vi "FileIO - Save ROI Results.vi"(11 "ROI Results":T1(array[cluster])) -> ()   [LabVIEW 2014]
uses:
  TypeDef - File Actions.ctl
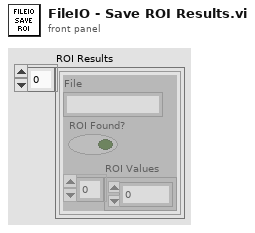
[diagram p1: front panel]
types:
  T1 = cluster{"File":string, "ROI Found?":bool, "ROI Values":dbl[]}[]
  T2 = typedef "TypeDef - File Actions.ctl" = enum16{"Read", "Write", "Get Current"}
  T3 = typedef "TypeDef - System Configuration.ctl" = cluster{"Results FilePath":path, "Analysis Parameters":cluster{"Area":cluster{"Lower Value":dbl, "Upper Value":dbl}, "Circle Filter Radius":cluster{"Lower Value":sgl, "Upper Value":sgl}, "Edge Detection Threshold":u16}, "ROI Parameters":cluster{"ROI size (in Radius)":cluster{"Width":dbl, "Height":dbl}}}
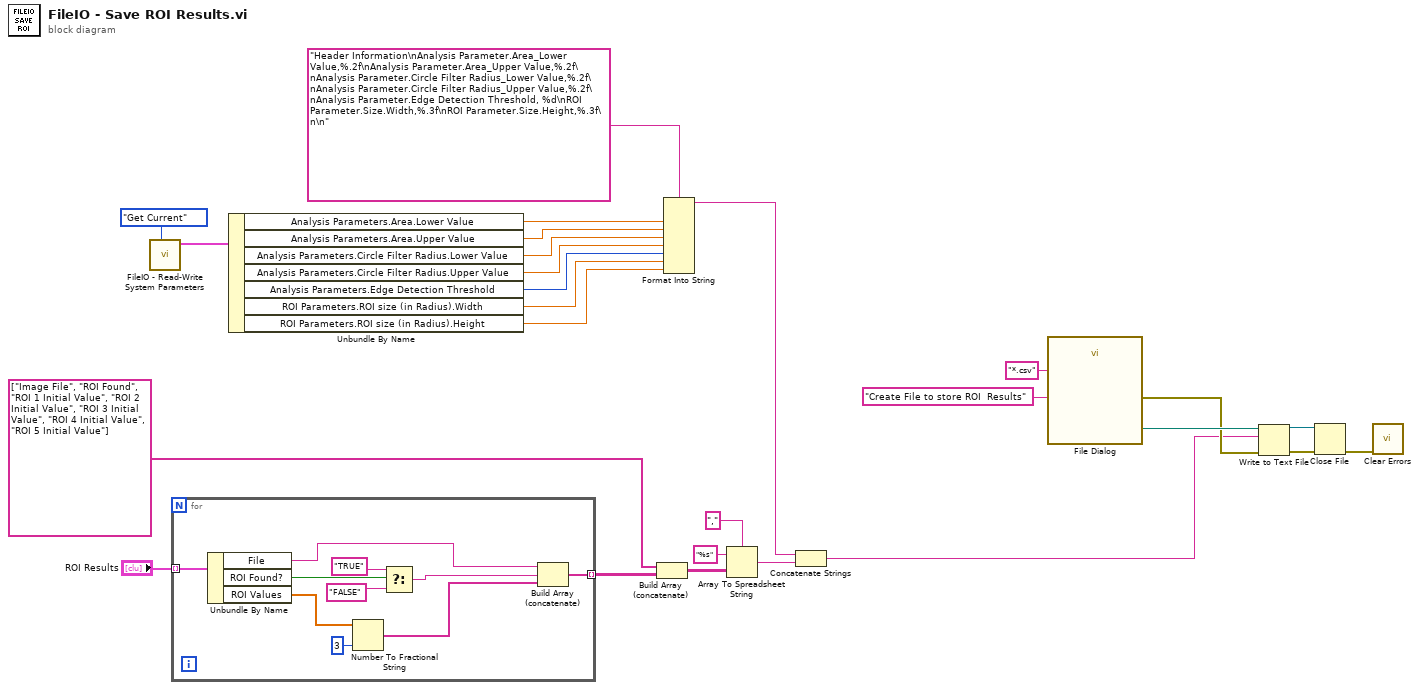
[diagram p0: block diagram]
diagram:
  n1 = call "FileIO - Read-Write System Parameters.vi"("Action"=TypeDef_-_File_Actions."Get Current") -> ("System Parameters out"=w12:T3)  [unwired: 9 in, 1 out]
  n2 = for {
    tunnel: "ROI Results" -> [w36] mode=indexing
    tunnel: [w28] -> w17 mode=indexing
    n3 = Unbundle By Name(w36) -> ("File"=w34:string, "ROI Found?"=w35:bool, "ROI Values"=w30:dbl[])
    n4 = Number To Fractional String(number=w30, precision (6)=i16 3) -> (F-format string=w29:string[])  [unwired: 2 in]
    n5 = Select(t="TRUE" ("File"), s=w35, f="FALSE" ("File")) -> (s? t:f=w31:string)
    n6 = Build Array (concatenate)(w34, w31, w29) -> (w28:string[])
  }
  n7 = Unbundle By Name(w12) -> ("Analysis Parameters.Area.Lower Value"=w9:dbl, "Analysis Parameters.Area.Upper Value"=w8:dbl, "Analysis Parameters.Circle Filter Radius.Lower Value"=w7:sgl, "Analysis Parameters.Circle Filter Radius.Upper Value"=w6:sgl, "Analysis Parameters.Edge Detection Threshold"=w5:u16, "ROI Parameters.ROI size (in Radius).Width"=w4:dbl, "ROI Parameters.ROI size (in Radius).Height"=w3:dbl)
  n8 = Build Array (concatenate)(string[] ["Image File", "ROI Found", "ROI 1 Initial Value", "ROI 2 Initial Value", "ROI 3 Initial Value", "ROI 4 Initial Value", "ROI 5 Initial Value"], w17) -> (w16:string[][])
  n9 = Format Into String(format string="Header Information\nAnalysis Parameter.Area_Lower Value,%.2f\nAnalysis Parameter.Area_Upper Value,%.2f\nAnalysis Parameter.Circle Filter Radius_Lower Value,%.2f\nAnalysis Parameter.Circle Filter Radius_Upper Value,%.2f\nAnalysis Parameter.Edge Detection Threshold, %d\nROI Parameter.Size.Width,%.3f\nROI Parameter.Size.Height,%.3f\n\n", w9, w8, w7, w6, w5, w4, w3) -> (resulting string=w1:string)  [unwired: 2 in, 1 out]
  n10 = Array To Spreadsheet String(delimiter (Tab)=",", array=w16, 3:"%s" ("format string")) -> (spreadsheet string=w11:string)
  n11 = Concatenate Strings(w1, w11) -> (w10:string)
  n12 = call "File Dialog"("prompt"="Create File to store ROI  Results", "pattern (all files)"="*.csv") -> ("selected path"=w20:path, "error out"=w19:errorcluster)  [unwired: 10 in, 2 out]
  n13 = Write to Text File(file (use dialog)=w20, text=w10, error in=w19) -> (refnum out=w22:refnum<file>, error out=w23:errorcluster)  [unwired: 1 in, 1 out]
  n14 = Close File(refnum=w22, error in=w23) -> (error out=w21:errorcluster)  [unwired: 1 out]
  n15 = call <vilib>:"Clear Errors.vi"("error in (no error)"=w21) -> ()  [unwired: 5 in, 2 out]
